vi "Temperature Warnings.vi"(8 "错误输入":cluster{"状态":bool, "代码":i32, "源":string}, 11 "气象数据输入":T1={"当前温度"=0.0, "最高温度"=0.0, "最低温度"=0.0, "温度警告？"=FALSE, "温度警告文本"="无警告", "当前风速"=0.0, "最大风速"=0.0, "风速警告？"=FALSE, "风速警告文本"="无警告"}) -> (0 "错误输出":cluster{"状态":bool, "代码":i32, "源":string}, 3 "气象数据输出":T1={"当前温度"=0.0, "最高温度"=0.0, "最低温度"=0.0, "温度警告？"=FALSE, "温度警告文本"="无警告", "当前风速"=0.0, "最大风速"=0.0, "风速警告？"=FALSE, "风速警告文本"="无警告"})   [LabVIEW 2012]
doc: "本VI用于判定基于当前温度值和边界设置的字符串，该字符串输出至气象站。"
uses:
  Weather Data.ctl
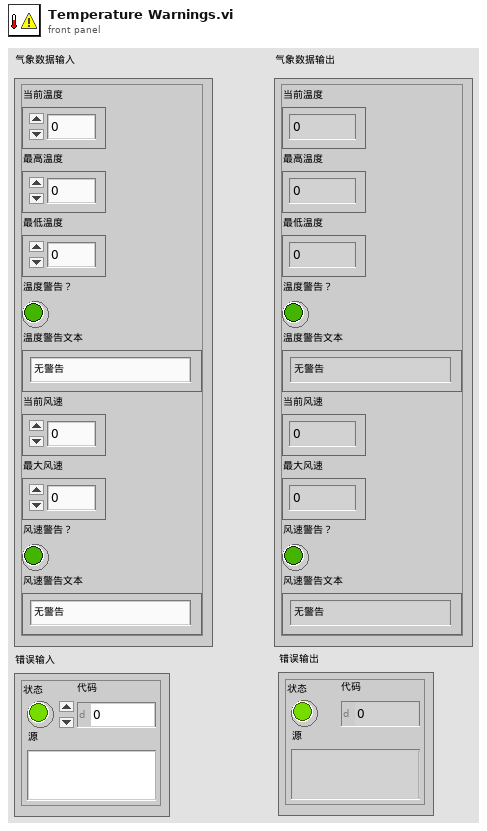
[diagram p1: front panel]
types:
  T1 = typedef "Weather Data.ctl" = cluster{"当前温度":dbl, "最高温度":dbl, "最低温度":dbl, "温度警告？":bool, "温度警告文本":string, "当前风速":dbl, "最大风速":dbl, "风速警告？":bool, "风速警告文本":string}
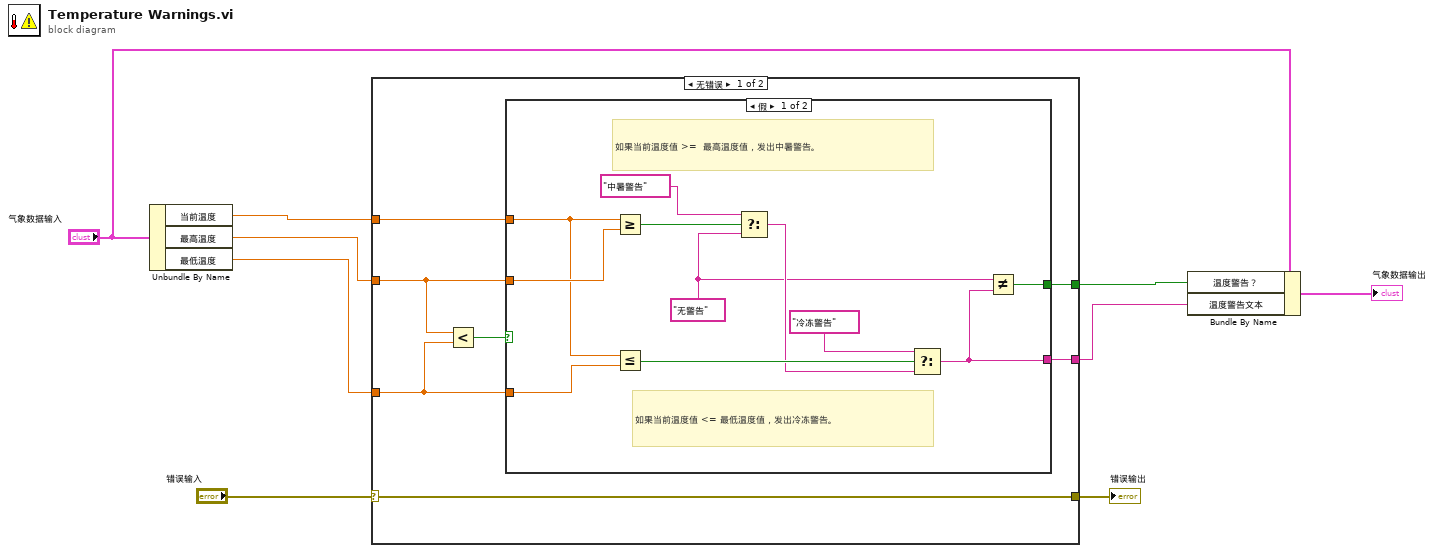
[diagram p0: block diagram]
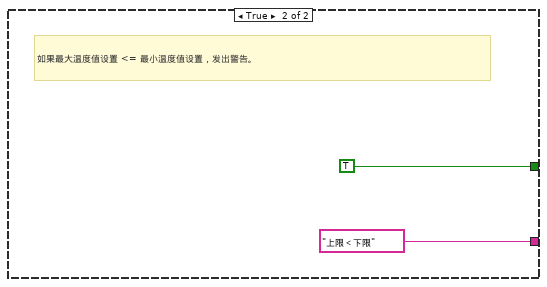
[diagram p2: hidden frame]
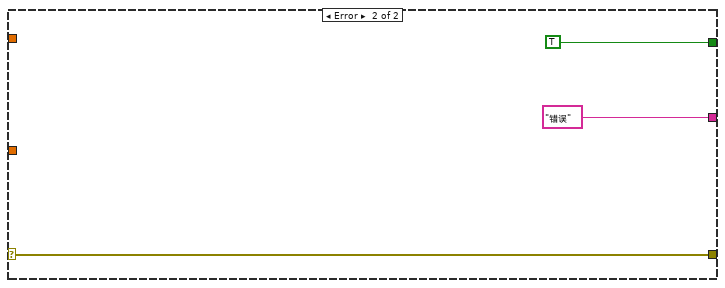
[diagram p3: hidden frame]
diagram:
  n1 = Unbundle By Name ("按名称解除捆绑")("气象数据输入") -> ("当前温度"=w7:dbl, "最高温度"=w6:dbl, "最低温度"=w5:dbl)
  n2 = case shown="无错误" "错误输入" {
    selector: "错误输入" -> [w14 w32]
    tunnel: [w16 "错误" ("f")] -> w4
    tunnel: [w15 TRUE] -> w3
    tunnel: [w14 w32] -> w8
    tunnel: w5 -> [w11 _]
    tunnel: w7 -> [w13 _]
    tunnel: w6 -> [w12 _]
    frame No Error {
      n3 = Less? ("小于？")(x=w12, y=w11) -> (x < y?=w10:bool)
      n4 = case shown="假" w10 {
        tunnel: [w17 "上限＜下限" ("f")] -> w16
        tunnel: [w27 TRUE] -> w15
        tunnel: w12 -> [w26 _]
        tunnel: w11 -> [w23 _]
        tunnel: w13 -> [w19 _]
        frame False {
          w18 = "无警告" ("f")
          # "如果当前温度值 <= 最低温度值，发出冷冻警告。"
          # "如果当前温度值 >=  最高温度值，发出中暑警告。"
          n5 = Greater Or Equal? ("大于等于？")(x=w19, y=w26) -> (x >= y?=w25:bool)
          n6 = Less Or Equal? ("小于等于？")(x=w19, y=w23) -> (x <= y?=w21:bool)
          n7 = Select ("选择")(t="中暑警告", s=w25, f=w18) -> (s? t:f=w20:string)
          n8 = Select ("选择")(t="冷冻警告", s=w21, f=w20) -> (s? t:f=w17:string)
          n9 = Not Equal? ("不等于？")(x=w18, y=w17) -> (x != y?=w27:bool)
        }
        frame True {
          # "如果最大温度值设置 <= 最小温度值设置，发出警告。"
        }
      }
    }
    frame Error {
    }
  }
  "错误输出" <- w8
  n10 = Bundle By Name ("按名称捆绑")(cluster="气象数据输入", "温度警告？"=w3, "温度警告文本"=w4) -> (→"气象数据输出":T1)
